vi "provide_note_book_info.vi"(8 "error in (no error)":errorcluster, 10 "notebook string in":string, 11 "GenericPlugin in":refnum<class "ImagingModeTS090821Circular2D.lvclass">) -> (0 "error out":errorcluster, 2 "notebook string out":string, 3 "GenericPlugin out":refnum<class "ImagingModeTS090821Circular2D.lvclass">)   [LabVIEW 2010, in "ImagingModeTS090821Circular2D.lvclass"]
uses:
  ImagingModeTS090821Circular2D.lvclass
  ImagingModeDL091001Scaffold/ImagingModeDL091001Scaffold/ImagingModeDL091001Scaffold.lvclass
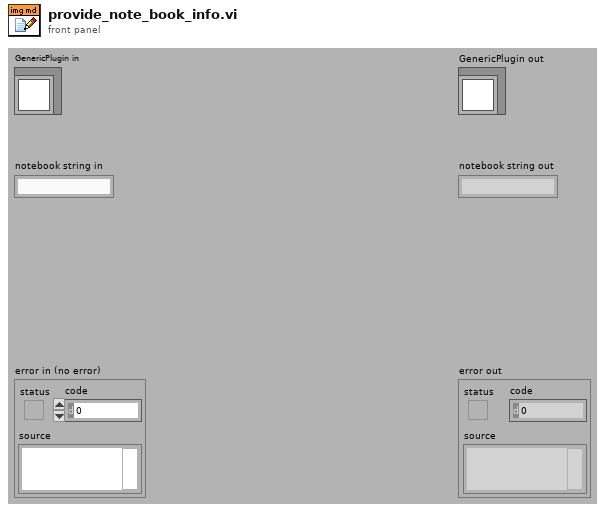
[diagram p1: front panel]
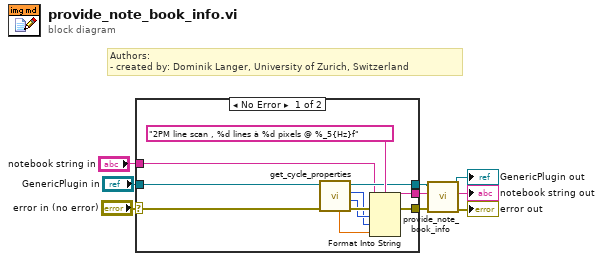
[diagram p0: block diagram]
diagram:
  # "Authors: \n- created by: Dominik Langer, University of Zurich, Switzerland"
  n1 = case shown="No Error" "error in (no error)" {
    selector: "error in (no error)" -> [w19 w23]
    tunnel: "notebook string in" -> [w11 w21]
    tunnel: "GenericPlugin in" -> [w18 w22]
    tunnel: [w13 w23] -> w6
    tunnel: [w12 w22] -> w5
    tunnel: [w10 w21] -> w4
    frame No Error {
      n2 = call-dynamic "get_cycle_properties.vi"("error in (no error)"=w19, "ScanModeTS090821Circular2D in"=w18) -> ("error out"=w17:errorcluster, "number of cycles"=w15:i32, "total number of pixels per cycle"=w14:i32, "ScanModeTS090821Circular2D out"=w12:refnum<class "ImagingModeTS090821Circular2D.lvclass">, "scan rate"=w16:dbl[unit])  [unwired: 3 in, 2 out]
      n3 = Format Into String(format string="2PM line scan , %d lines à %d pixels @ %_5{Hz}f", initial string=w11, error in=w17, w15, w14, w16) -> (resulting string=w10:string, error out=w13:errorcluster)
    }
    frame Error {
    }
  }
  n4 = call-parent "provide_note_book_info.vi"("error in (no error)"=w6, "notebook string in"=w4, "GenericPlugin in"=w5) -> ("error out"=→"error out":errorcluster, "notebook string out"=→"notebook string out":string, "GenericPlugin out"=→"GenericPlugin out":refnum<class "ImagingModeTS090821Circular2D.lvclass">)  [unwired: 6 in]
